vi "random_array_2D.vi"(10 "x":i32=8, 11 "y":i32=8) -> (2 "array":i16[][](array[numeric]))   [LabVIEW 2013]
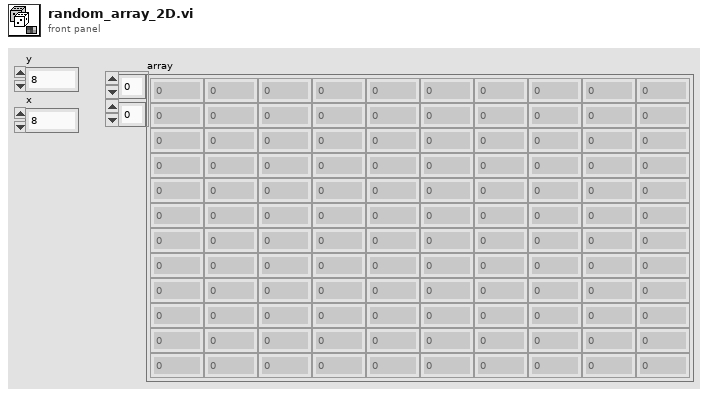
[diagram p1: front panel]
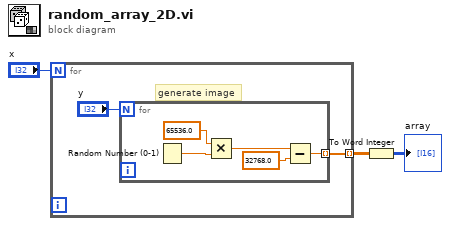
[diagram p0: block diagram]
diagram:
  n1 = for {
    N: "x" -> [_]
    tunnel: [w4] -> w2 mode=indexing
    # "generate image"
    n2 = for {
      N: "y" -> [_]
      tunnel: [w6] -> w4 mode=indexing
      n3 = Random Number (0-1)() -> (number: 0 to 1=w10:dbl)
      n4 = Multiply(x=65536.0, y=w10) -> (x*y=w8:dbl)
      n5 = Subtract(x=w8, y=32768.0) -> (x-y=w6:dbl)
    }
  }
  n6 = To Word Integer(number=w2) -> (16bit integer=→"array":i16[][])
